vi "Fetch Max Min Waveform.vi"(4 "Sparsing (0: Every point)":i32, 5 "Number of points (0: All points)":i32, 7 "First point (0: First point)":i32, 8 "error in (no error)":errorcluster, 9 "Timeout (10000 ms)":u32=10000, 10 "Source (0: Channel 1)":u16(ring) items=["Channel 1", "Channel 2", "Channel 3", "Channel 4", "Memory 1", "Memory 2", "Memory 3", "Memory 4", "Function 1", "Function 2", "Function 3", "Function 4", "Function 5", "Function 6", "Function 7", "Function 8"], 11 "VISA resource name":refnum<visa-resource-name>) -> (0 "error out":errorcluster, 1 "Min":waveform(dbl)(graph), 2 "Max":waveform(dbl)(graph), 3 "VISA resource name out":refnum<visa-resource-name>)   [LabVIEW 2013, in "LeCroy Wave Series.lvlib"]
doc: "Returns the two waveforms the oscilloscope acquired for the specified channel. The waveforms are from an acquisition that you initiate prior to calling this VI. A both waveforms must be in one channel together. It is usable for math functions, for example math function envelope get two waveforms. One is roof and second is floor.\n\nYou use the Initiate VI to start an acquisition on the channels that you enable with the <B>Configure Channel</B> VI. The oscilloscope acquires waveforms for the enabled channels concurrently. You must call this VI separately for each enabled channel to obtain the waveforms.\n\n<B>Note</B> This VI does not check the instrument status. Typically, you call this VI only in a sequence of calls to other low-level instrument driver VIs. The sequence performs one operation. You use the low-level VIs to optimize one or more aspects of interaction with the instrument."
uses:
  LeCroy Wave Series.lvlib
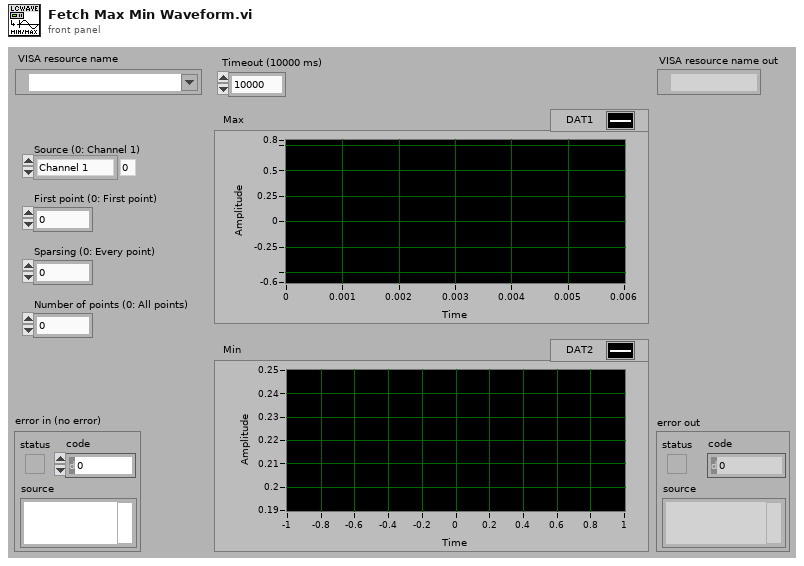
[diagram p1: front panel]
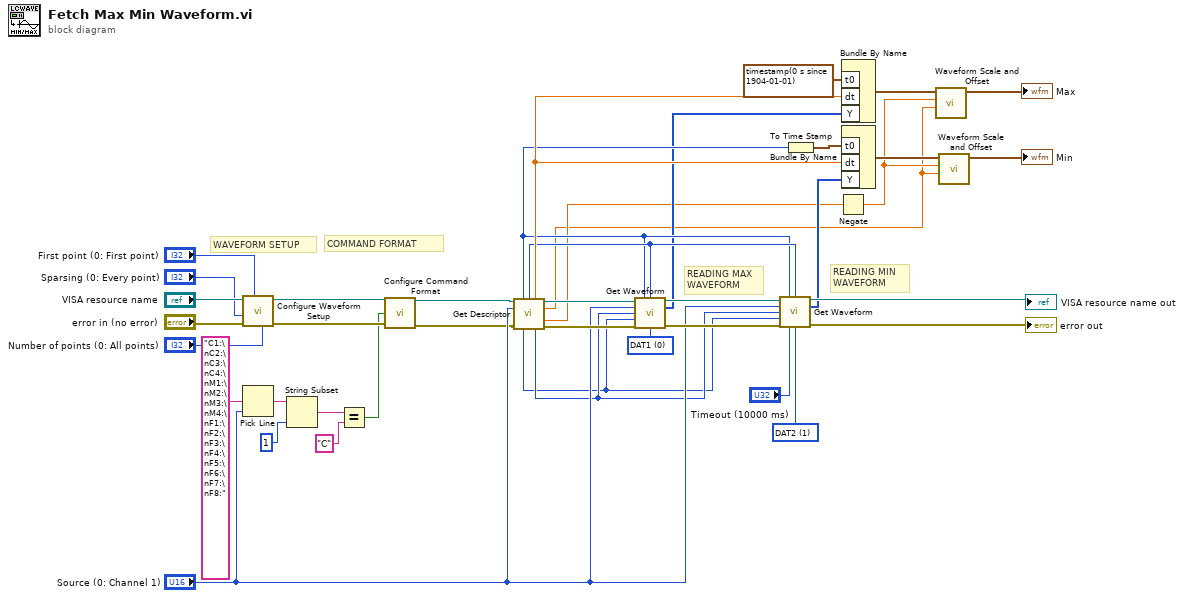
[diagram p0: block diagram]
diagram:
  w16 = u16 1 items=["DAT1", "DAT2"] ("Array (1: DAT1)")
  w17 = u16 0 items=["DAT1", "DAT2"] ("Array (1: DAT1)")
  # "READING MIN WAVEFORM"
  # "READING MAX WAVEFORM"
  # "WAVEFORM SETUP"
  # "COMMAND FORMAT"
  n1 = call "Configure Waveform Setup.vi"("Number of points (0: All points)"="Number of points (0: All points)", "First point (0: First point)"="First point (0: First point)", "error in (no error)"="error in (no error)", "Sparsing (0: Every point)"="Sparsing (0: Every point)", "VISA resource name"="VISA resource name") -> ("error out"=w31:errorcluster, "VISA resource name out"=w32:refnum<visa-resource-name>)  [unwired: 5 in]
  n2 = Pick Line(multi-line string="C1:\nC2:\nC3:\nC4:\nM1:\nM2:\nM3:\nM4:\nF1:\nF2:\nF3:\nF4:\nF5:\nF6:\nF7:\nF8:", line index="Source (0: Channel 1)") -> (output string=w38:string)  [unwired: 1 in]
  n3 = String Subset(string=w38, length (rest)=1 ("offset (0)")) -> (substring=w36:string)  [unwired: 1 in]
  n4 = Equal?(x=w36, y="C") -> (x = y?=w30:bool)
  n5 = call "Configure Command Format.vi"("VISA resource name"=w32, "Command format (T: Byte)"=w30, "error in (no error)"=w31) -> ("VISA resource name out"=w3:refnum<visa-resource-name>, "error out"=w2:errorcluster)  [unwired: 11 in]
  n6 = call "Get Descriptor.vi"("VISA resource name"=w3, "Source (0: Channel 1)"="Source (0: Channel 1)", "error in (no error)"=w2) -> ("First Valid Point"=w13:i32, "Last Valid Point"=w14:i32, "Horizontal interval"=w18:sgl, "VISA resource name out"=w41:refnum<visa-resource-name>, "Vertical gain"=w4:sgl, "Vertical offset"=w6:sgl, "Number Of Data Points"=w15:i32, "Command type"=w24:i16, "error out"=w40:errorcluster)  [unwired: 2 in, 2 out]
  n7 = call "Get Waveform.vi"("VISA resource name"=w41, "First Valid Point"=w13, "Last Valid Point"=w14, "Source (0: Channel 1)"="Source (0: Channel 1)", "Command type (0: byte)"=w24, "Number Of Data Points (10000)"=w15, "error in (no error)"=w40, "Array (0: DAT1)"=w17) -> ("VISA resource name out"=w29:refnum<visa-resource-name>, "Waveform Graph"=w11:i16[], "error out"=w27:errorcluster)  [unwired: 5 in]
  n8 = call "Get Waveform.vi"("VISA resource name"=w29, "First Valid Point"=w13, "Last Valid Point"=w14, "Source (0: Channel 1)"="Source (0: Channel 1)", "Command type (0: byte)"=w24, "Number Of Data Points (10000)"=w15, "error in (no error)"=w27, "Timeout (10000 ms)"="Timeout (10000 ms)", "Array (0: DAT1)"=w16) -> ("VISA resource name out"=→"VISA resource name out":refnum<visa-resource-name>, "Waveform Graph"=w12:i16[], "error out"=→"error out":errorcluster)  [unwired: 4 in]
  n9 = To Time Stamp(1:w13) -> (0:w23:timestamp)
  n10 = Negate(x=w6) -> (-x=w5:sgl)
  n11 = Bundle By Name ("Build Waveform")("t0"=timestamp(0 s since 1904-01-01), "dt"=w18, "Y"=w11) -> (w10:waveform(i16))  [unwired: 1 in]
  n12 = Bundle By Name ("Build Waveform")("t0"=w23, "dt"=w18, "Y"=w12) -> (w8:waveform(i16))  [unwired: 1 in]
  n13 = call <vilib>:"Waveform Scale and Offset.vi"("scale"=w4, "offset"=w5, "waveform in"=w10) -> ("waveform out"=→"Max":waveform(dbl))  [unwired: 7 in, 1 out]
  n14 = call <vilib>:"Waveform Scale and Offset.vi"("scale"=w4, "offset"=w5, "waveform in"=w8) -> ("waveform out"=→"Min":waveform(dbl))  [unwired: 7 in, 1 out]
